vi "wait for available bytes at serial port.vi"(8 "error in (no error)":errorcluster, 10 "ms to wait":u32, 11 "VISA resource name":refnum<visa-resource-name>) -> (0 "error out":errorcluster, 1 "bytes available":u32, 3 "VISA resource name 2":refnum<visa-resource-name>)   [LabVIEW 2013]
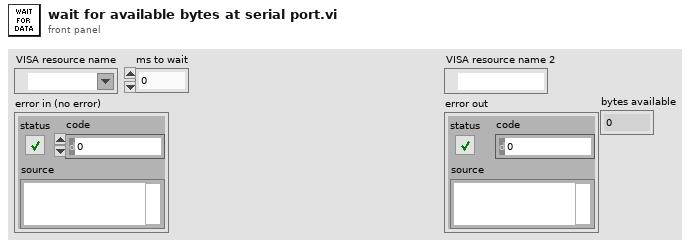
[diagram p1: front panel]
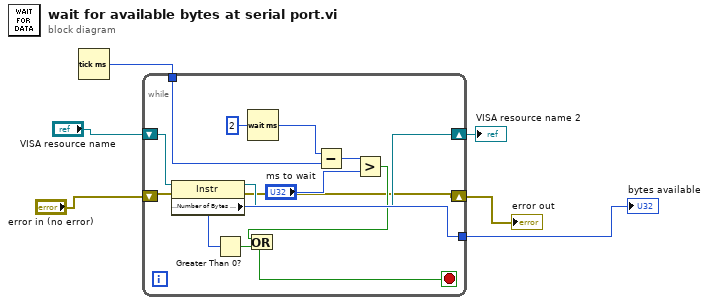
[diagram p0: block diagram]
diagram:
  n1 = Tick Count (ms)() -> (millisecond timer value=w1:u32)
  n2 = while {
    shift-right: [w7] -> w3
    shift-left: "error in (no error)" -> [w8]
    shift-right: [w9] -> w4
    shift-left: "VISA resource name" -> [w19]
    tunnel: [w17] -> w2
    tunnel: w1 -> [w13]
    stop <- w16 stop-if-true
    n3 = property class="Instr"(reference=w19, error in=w8) -> (reference out=w9:refnum<visa-resource-name>, error out=w7:errorcluster, "Serial Settings:Number of Bytes at Serial Port"=w17:u32)
    n4 = Greater Than 0?(x=w17) -> (x > 0?=w18:bool)
    n5 = Wait (ms)(milliseconds to wait=u32 2) -> (millisecond timer value=w14:u32)
    n6 = Subtract(x=w14, y=w13) -> (x-y=w12:u32)
    n7 = Greater?(x=w12, y="ms to wait") -> (0:w10:bool)
    n8 = Or(x=w10, y=w18) -> (x .or. y?=w16:bool)
  }
  "VISA resource name 2" <- w4
  "error out" <- w3
  "bytes available" <- w2
